vi "ABB Test personel.vi"() -> (2 "Attendance data":string[][](array[string]), 3 "Personel out":string[](array[string]))   [LabVIEW 2017]
uses:
  ABB global.vi
panel:
  in  "Company":string[](array[string])
  in  "Attendees":string[](array[string])
  in  "No. Attendees":i32(ring) items=["None", "1", "2", "3", "4", "5", "6"]
  out "Current Date":string
  in  "Use current date":bool
  in  "Date":string
  in  "Approved by":u16(ring)
  in  "Tested By":u16(ring)
  in  "Exit":bool
  # "Test Personnel"
  # "Attendance"
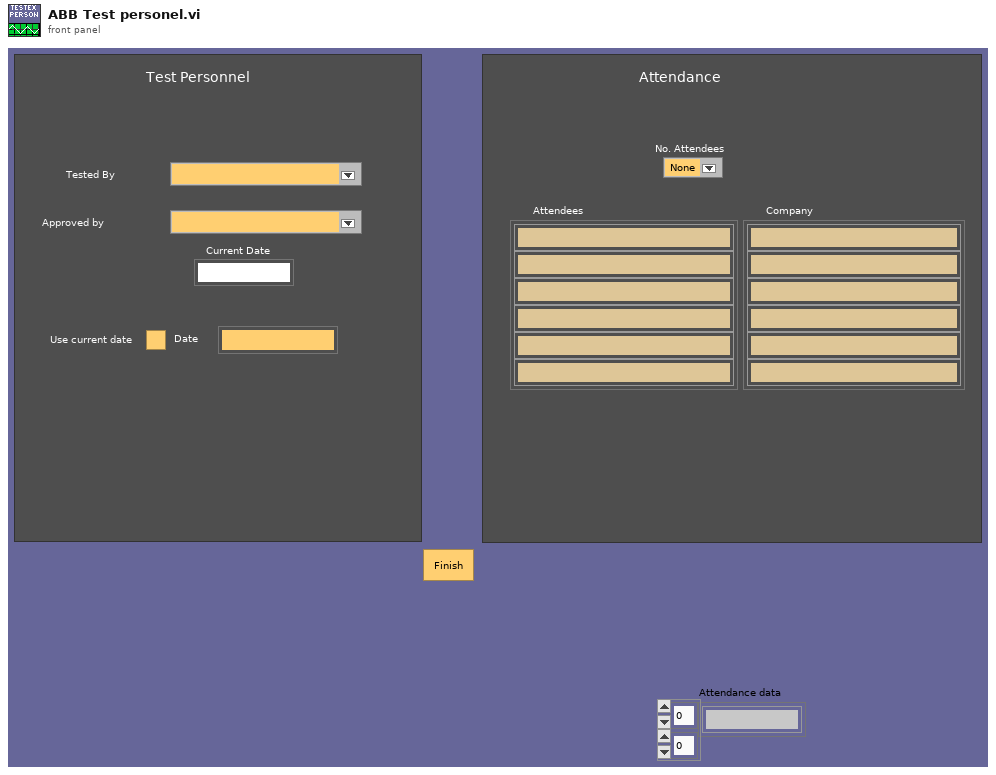
[diagram p1: front panel]
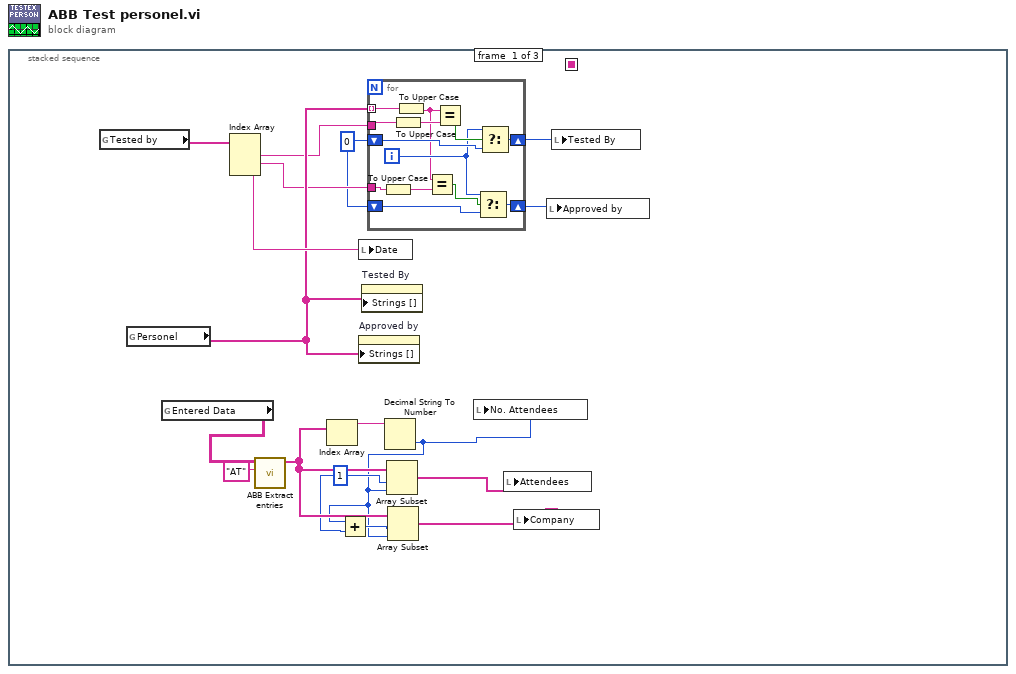
[diagram p0: block diagram]
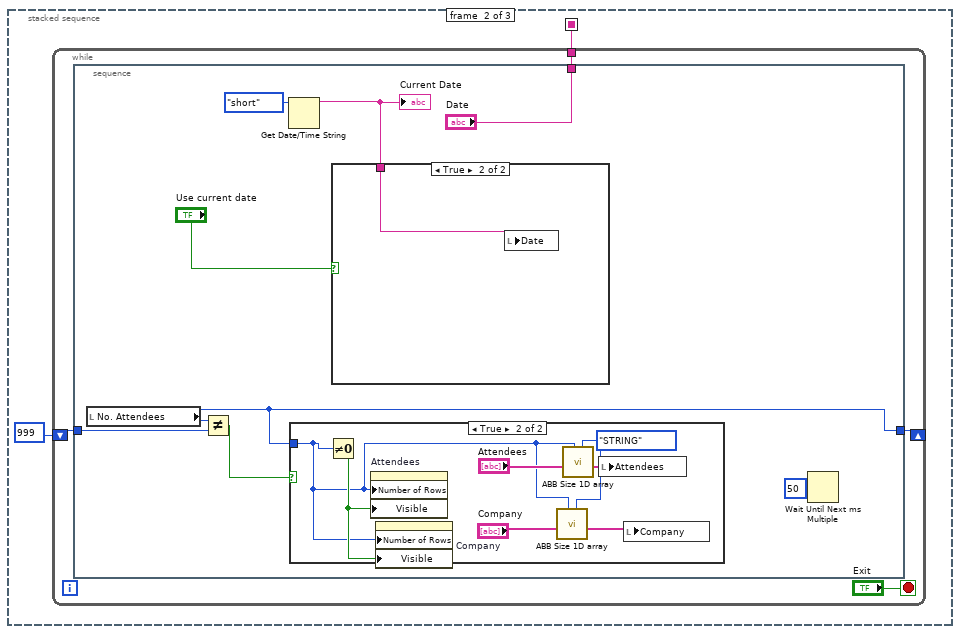
[diagram p2: hidden frame]
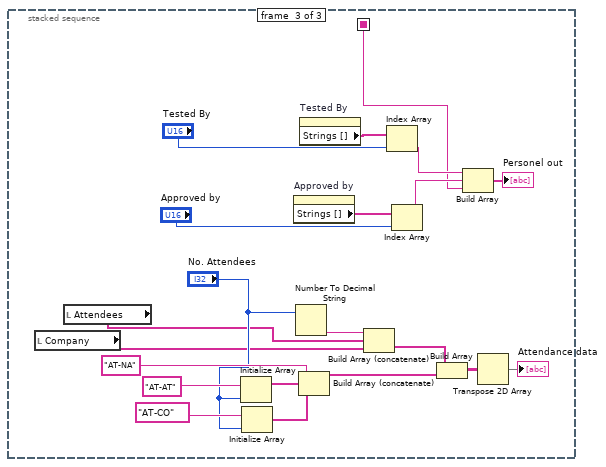
[diagram p5: hidden frame]
diagram:
  n1 = stacked-sequence {
    seq-local: [_ w32 _] -> [_ _ w67]
    frame #0 {
      w6 = 1 ("index")
      w11 = 0
      n2 = global read "ABB global.vi" "Tested by"() -> (w17:string[])
      n3 = global read "ABB global.vi" "Personel"() -> (w15:string[])
      n4 = global read "ABB global.vi" "Entered Data"() -> (w8:string[][])
      n5 = Index Array(array=w17) -> (element #1=w14:string, element #2=w12:string, element #3=w16:string)  [unwired: 3 in]
      n6 = call "ABB Extract entries.vi"("Entry ID"="AT", "Entry table in"=w8) -> ("Selected Entries"=w7:string[])  [unwired: 9 in]
      n7 = Index Array(array=w7) -> (element=w10:string)  [unwired: 1 in]
      n8 = local write "Date"(w16) -> ()
      n9 = property on="Approved by" class="Ring (strict)"("Strings []"=w15) -> ()  [unwired: 2 in, 2 out]
      n10 = property on="Tested By" class="Ring (strict)"("Strings []"=w15) -> ()  [unwired: 2 in, 2 out]
      n11 = for {
        tunnel: w15 -> [w30] mode=indexing
        tunnel: w14 -> [w29]
        shift-right: [w25] -> w13
        shift-left: w11 -> [w27]
        tunnel: w12 -> [w24]
        shift-right: [w18] -> w1
        shift-left: w11 -> [w23]
        i -> [w22]
        n12 = To Upper Case(1:w24) -> (0:w21:string)
        n13 = To Upper Case(1:w29) -> (0:w28:string)
        n14 = To Upper Case(1:w30) -> (0:w20:string)
        n15 = Equal?(x=w20, y=w21) -> (x = y?=w19:bool)
        n16 = Equal?(x=w20, y=w28) -> (x = y?=w26:bool)
        n17 = Select(t=w22, s=w19, f=w23) -> (s? t:f=w18:i32)
        n18 = Select(t=w22, s=w26, f=w27) -> (s? t:f=w25:i32)
      }
      n19 = Decimal String To Number(string=w10) -> (number=w3:i32)  [unwired: 2 in, 1 out]
      n20 = Add(x=w3, y=w6) -> (x+y=w5:i32)
      n21 = Array Subset(array=w7, index=w6, length=w3) -> (w2:string[])
      n22 = Array Subset(array=w7, index=w5, length=w3) -> (w4:string[])
      n23 = local write "No. Attendees"(w3) -> ()
      n24 = local write "Attendees"(w2) -> ()
      n25 = local write "Company"(w4) -> ()
      n26 = local write "Approved by"(w1) -> ()
      n27 = local write "Tested By"(w13) -> ()
    }
    frame #1 {
      n28 = while {
        tunnel: [w35] -> w32
        shift-right: [w33] -> _
        shift-left: 999 -> [w34]
        stop <- "Exit" stop-if-true
        n29 = stacked-sequence {
          tunnel: ["Date"] -> w35
          tunnel: w34 -> [w39]
          tunnel: [w37] -> w33
          frame #0 {
            n30 = local read "No. Attendees"() -> (w37:i32)
            n31 = Not Equal?(x=w37, y=w39) -> (x != y?=w38:bool)
            n32 = Get Date/Time String(date format (0)=enum16{"short", "long", "abbreviated"}."short") -> (date string=w40:string)  [unwired: 2 in, 1 out]
            "Current Date" <- w40
            n33 = case shown="True" w38 {
              tunnel: w37 -> [_ w47]
              frame False {
              }
              frame True {
                w46 = enum16{"Integer", "DBL", "STRING", "BOOLEAN"}."STRING" ("Type")
                n34 = Not Equal To 0?(x=w47) -> (x != 0?=w51:bool)
                n35 = property on="Attendees" class="Arr (strict)"("Number of Rows"=w47, "Visible"=w51) -> ()  [unwired: 2 in, 2 out]
                n36 = property on="Company" class="Arr (strict)"("Number of Rows"=w47, "Visible"=w51) -> ()  [unwired: 2 in, 2 out]
                n37 = call "ABB Size 1D array.vi"("Type"=w46, "Size"=w47, "String Array in"="Company") -> ("String Array out"=w48:string[])  [unwired: 5 in, 3 out]
                n38 = call "ABB Size 1D array.vi"("Type"=w46, "Size"=w47, "String Array in"="Attendees") -> ("String Array out"=w45:string[])  [unwired: 5 in, 3 out]
                n39 = local write "Attendees"(w45) -> ()
                n40 = local write "Company"(w48) -> ()
              }
            }
            n41 = case shown="True" "Use current date" {
              tunnel: w40 -> [_ w52]
              frame False {
              }
              frame True {
                n42 = local write "Date"(w52) -> ()
              }
            }
            n43 = Wait Until Next ms Multiple(millisecond multiple=u32 50) -> ()  [unwired: 1 out]
          }
        }
      }
    }
    frame #2 {
      n44 = local read "Company"() -> (w53:string[])
      n45 = local read "Attendees"() -> (w54:string[])
      n46 = Initialize Array("AT-AT", "No. Attendees") -> (w62:string[])
      n47 = Initialize Array("AT-CO", "No. Attendees") -> (w56:string[])
      n48 = property on="Approved by" class="Ring (strict)"() -> ("Strings []"=w71:string[])  [unwired: 2 in, 2 out]
      n49 = Number To Decimal String(number="No. Attendees") -> (decimal integer string=w65:string)  [unwired: 1 in]
      n50 = Build Array (concatenate)("AT-NA", w62, w56) -> (w60:string[])
      n51 = property on="Tested By" class="Ring (strict)"() -> ("Strings []"=w73:string[])  [unwired: 2 in, 2 out]
      n52 = Build Array (concatenate)(w65, w54, w53) -> (w61:string[])
      n53 = Index Array(array=w73, index="Tested By") -> (element=w69:string)
      n54 = Index Array(array=w71, index="Approved by") -> (element=w68:string)
      n55 = Build Array(w61, w60) -> (w59:string[][])
      n56 = Build Array(w69, w68, w67) -> (→"Personel out":string[])
      n57 = Transpose 2D Array(2D array=w59) -> (transposed array=→"Attendance data":string[][])
    }
  }
